vi "PH_AccumCounts.vi"(0 "Data In":u32[](array[numeric]), 1 "Reset":bool, 5 "Data Count":i32, 11 "Acc X Overflows":i32=25) -> (4 "Histograms":i32[][](array[numeric]), 8 "Accum Counts":u32[](array[numeric]), 10 "Acc Time Ok":bool, 13 "Total Oveflow Count":u64, 14 "Num Records Total":i32)   [LabVIEW 8.6]
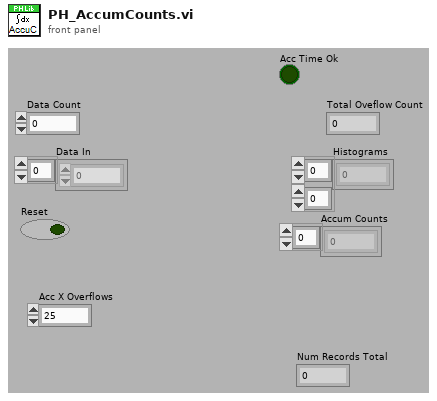
[diagram p1: front panel]
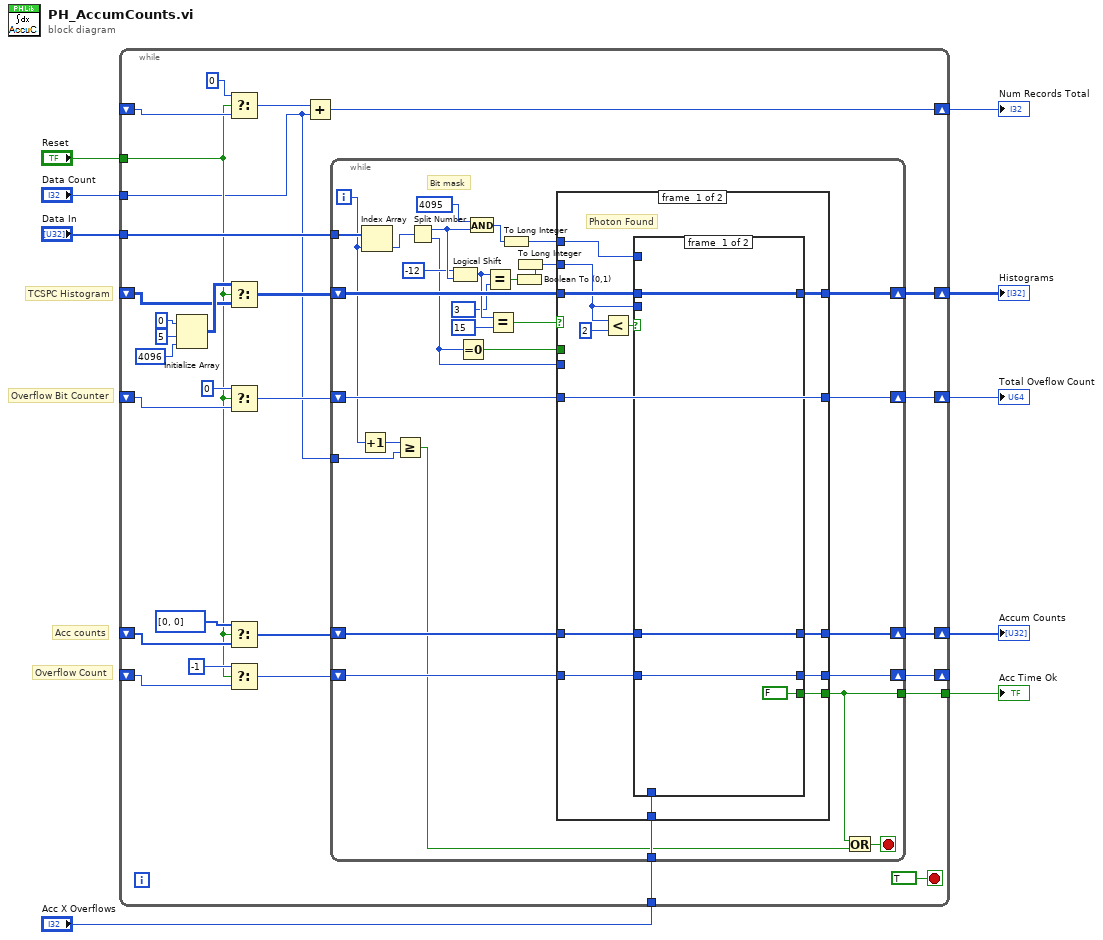
[diagram p0: block diagram]
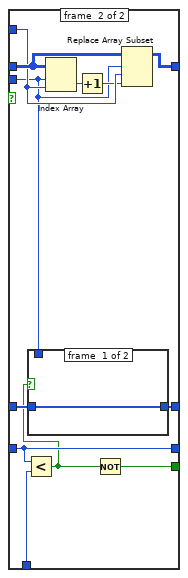
[diagram p2: hidden frame]
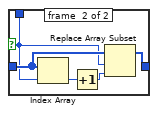
[diagram p3: hidden frame]
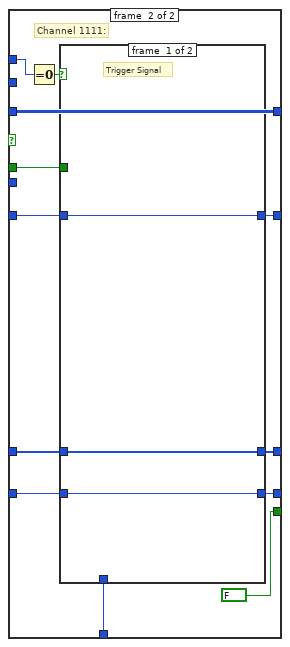
[diagram p4: hidden frame]
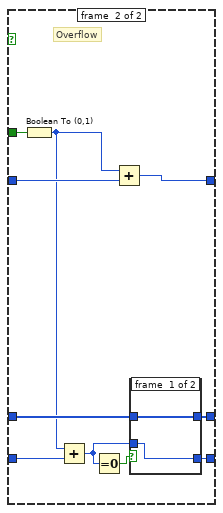
[diagram p5: hidden frame]
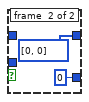
[diagram p6: hidden frame]
diagram:
  # "Overflow Count"
  # "Acc counts"
  # "TCSPC Histogram"
  # "Overflow Bit Counter"
  n1 = while {
    tunnel: "Data In" -> [w36]
    shift-right: [w37] -> w9
    shift-left: _ -> [w32]
    tunnel: "Reset" -> [w12]
    shift-right: [w29] -> w3
    shift-left: _ -> [w28]
    shift-right: [w26] -> w2
    shift-left: _ -> [w25]
    shift-right: [w23] -> _
    shift-left: _ -> [w22]
    tunnel: "Acc X Overflows" -> [w21]
    tunnel: "Data Count" -> [w11]
    shift-right: [w17] -> w4
    shift-left: _ -> [w19]
    tunnel: [w10] -> w1
    stop <- TRUE stop-if-true
    n2 = Initialize Array(0 ("element"), 5 ("dimension size"), 4096 ("dimension size")) -> (w33:i32[][])
    n3 = Select(t=0 ("Data Count 2"), s=w12, f=w19) -> (s? t:f=w18:i32)
    n4 = Select(t=w33, s=w12, f=w32) -> (s? t:f=w34:i32[][])
    n5 = Select(t=u64 0, s=w12, f=w28) -> (s? t:f=w30:u64)
    n6 = Select(t=u32[] [0, 0] ("initialized array"), s=w12, f=w25) -> (s? t:f=w27:u32[])
    n7 = Select(t=-1, s=w12, f=w22) -> (s? t:f=w24:i32)
    n8 = Add(x=w18, y=w11) -> (x+y=w17:i32)
    n9 = while {
      tunnel: w36 -> [w52]
      shift-right: [w65] -> w37
      shift-left: w34 -> [w67]
      shift-right: [w59] -> w29
      shift-left: w30 -> [w60]
      shift-right: [w56] -> w26
      shift-left: w27 -> [w57]
      shift-right: [w54] -> w23
      shift-left: w24 -> [w55]
      tunnel: w21 -> [w45]
      tunnel: w11 -> [w42]
      tunnel: [w39] -> w10
      i -> [w44]
      stop <- w40 stop-if-true
      # "Bit mask"
      n10 = Increment(x=w44) -> (x+1=w43:i32)
      n11 = Index Array(array=w52, index=w44) -> (element=w51:u32)
      n12 = Greater Or Equal?(x=w43, y=w42) -> (x >= y?=w41:bool)
      n13 = Split Number(x=w51) -> (hi(x)=w64:u16, lo(x)=w53:u16)
      n14 = Logical Shift(y=i8 -12, x=w64) -> (x << y=w50:u16)
      n15 = Equal To 0?(x=w53) -> (x = 0?=w58:bool)
      n16 = And(x=u16 4095, y=w64) -> (x .and. y?=w68:u16)
      n17 = Equal?(x=w50, y=u16 3) -> (x = y?=w48:bool)
      n18 = Equal?(x=w50, y=u16 15) -> (x = y?=w61:bool)
      n19 = To Long Integer(number=w68) -> (32bit integer=w66:i32)
      n20 = Boolean To (0,1)(Boolean=w48) -> (0, 1=w47:i16)
      n21 = To Long Integer(number=w47) -> (32bit integer=w46:i32)
      n22 = case shown="False" w61 {
        tunnel: w67 -> [w82 w113]
        tunnel: w66 -> [w79 w107]
        tunnel: [w81 w113] -> w65
        tunnel: w46 -> [w75 _]
        tunnel: w60 -> [w80 w115]
        tunnel: [w80 w114] -> w59
        tunnel: w58 -> [_ w112]
        tunnel: w57 -> [w78 w110]
        tunnel: [w77 w108] -> w56
        tunnel: w55 -> [w72 w111]
        tunnel: [w71 w109] -> w54
        tunnel: w53 -> [_ _]
        tunnel: w45 -> [w73 w106]
        tunnel: [w70 FALSE] -> w39
        frame #0 {
          # "Photon Found"
          n23 = Less?(x=w75, y=2) -> (x < y?=w76:bool)
          n24 = case shown="True" w76 {
            tunnel: w82 -> [w86 w98]
            tunnel: [w86 w97] -> w81
            tunnel: w79 -> [_ w96]
            tunnel: w75 -> [_ w91]
            tunnel: w78 -> [w85 w95]
            tunnel: [w85 w94] -> w77
            tunnel: w73 -> [_ w90]
            tunnel: w72 -> [w84 w89]
            tunnel: [w84 w89] -> w71
            tunnel: [FALSE w87] -> w70
            frame #0 {
            }
            frame #1 {
              n25 = Less?(x=w89, y=w90) -> (x < y?=w88:bool)
              n26 = case shown="True" w88 {
                tunnel: w95 -> [w99 w104]
                tunnel: [w99 w103] -> w94
                tunnel: w91 -> [_ w100]
                frame #0 {
                }
                frame #1 {
                  n27 = Index Array(array=w104, index=w100) -> (element=w102:u32)
                  n28 = Increment(x=w102) -> (x+1=w101:u32)
                  n29 = Replace Array Subset(array=w104, new element=w101, index=w100) -> (w103:u32[])
                }
              }
              n30 = Index Array(array=w98, index (row)=w91, index (col)=w96) -> (element=w93:i32)
              n31 = Increment(x=w93) -> (x+1=w92:i32)
              n32 = Not(x=w88) -> (.not. x?=w87:bool)
              n33 = Replace Array Subset(array=w98, new element=w92, index (row)=w91, index (col)=w96) -> (w97:i32[][])
            }
          }
        }
        frame #1 {
          # "Channel 1111:"
          n34 = Equal To 0?(x=w107) -> (x = 0?=w116:bool)
          n35 = case shown="True" w116 {
            tunnel: w115 -> [w119 w129]
            tunnel: [w119 w128] -> w114
            tunnel: w112 -> [_ w120]
            tunnel: w111 -> [w118 w123]
            tunnel: w110 -> [w117 w125]
            tunnel: [w118 w126] -> w109
            tunnel: [w117 w124] -> w108
            tunnel: w106 -> [_ _]
            frame #0 {
              # "Trigger Signal"
            }
            frame #1 {
              # "Overflow"
              n36 = Boolean To (0,1)(Boolean=w120) -> (0, 1=w121:i16)
              n37 = Add(x=w121, y=w123) -> (x+y=w122:i32)
              n38 = Equal To 0?(x=w122) -> (x = 0?=w127:bool)
              n39 = Add(x=w121, y=w129) -> (x+y=w128:u64)
              n40 = case shown="True" w127 {
                tunnel: w122 -> [w131 _]
                tunnel: [w131 0] -> w126
                tunnel: w125 -> [w130 _]
                tunnel: [w130 u32[] [0, 0] ("initialized array")] -> w124
                frame #0 {
                }
                frame #1 {
                }
              }
            }
          }
        }
      }
      n41 = Or(x=w39, y=w41) -> (x .or. y?=w40:bool)
    }
  }
  "Histograms" <- w9
  "Num Records Total" <- w4
  "Total Oveflow Count" <- w3
  "Accum Counts" <- w2
  "Acc Time Ok" <- w1
